vi "Actor Shutdown.vi"(8 "error in (no error)":errorcluster, 11 "IED in":refnum<class "IED.lvclass">) -> (0 "error out":errorcluster, 3 "IED out":refnum<class "IED.lvclass">)   [LabVIEW 2015, in "IED Actor.lvlib" / "IED.lvclass"]
doc: "This VI stops nested actors and sends success or failure to the SCADA Core."
uses:
  IED.lvclass
  IED.lvclass/IED.ctl
  <vilib>/ActorFramework/Message Enqueuer/Message Enqueuer.lvclass/Message Enqueuer.ctl
  <vilib>/ActorFramework/Message Enqueuer/Enqueue.vi
  <vilib>/ActorFramework/Message Priority Queue/Priority Enqueue.vi
  <vilib>/ActorFramework/Stop Msg/Stop Msg.lvclass
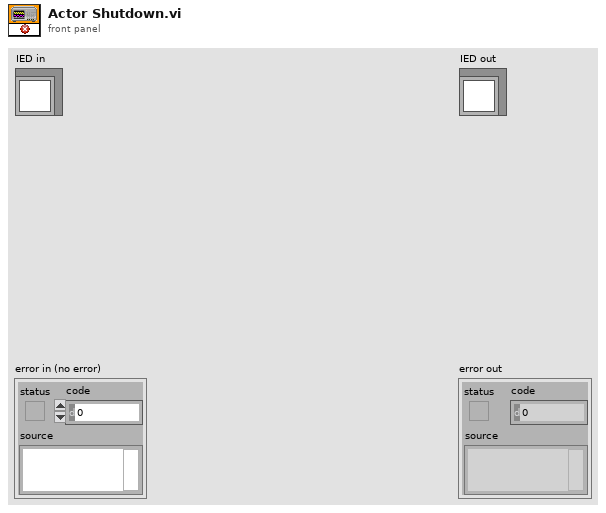
[diagram p1: front panel]
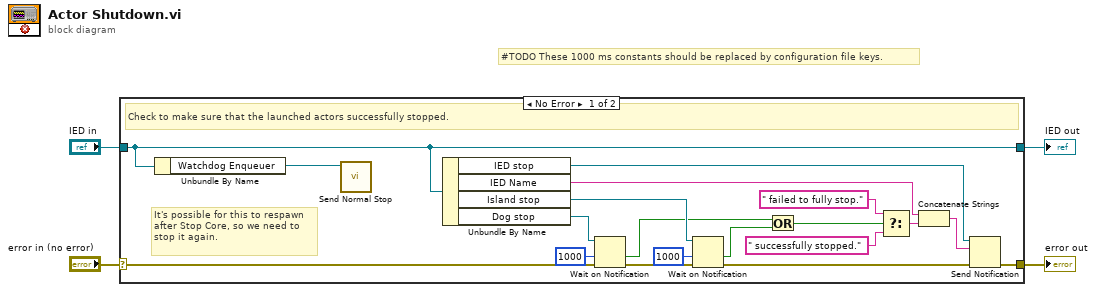
[diagram p0: block diagram]
diagram:
  # "#TODO These 1000 ms constants should be replaced by configuration file keys."
  n1 = case shown="No Error" "error in (no error)" {
    selector: "error in (no error)" -> [w23 w25]
    tunnel: [w14 w25] -> w3
    tunnel: [w6 w24] -> w1
    tunnel: "IED in" -> [w6 w24]
    frame No Error {
      # "It's possible for this to respawn after Stop Core, so we need to stop it again."
      # "Check to make sure that the launched actors successfully stopped."
      n2 = Unbundle By Name(w6) -> ("Watchdog Enqueuer"=w5:refnum<class "Message Enqueuer.lvclass">)
      n3 = call <vilib>:"Send Normal Stop.vi"("Message Enqueuer"=w5) -> ()  [unwired: 10 in, 1 out]
      n4 = Unbundle By Name(w6) -> ("IED stop"=w13:refnum<notifier>, "IED Name"=w8:string, "Island stop"=w19:refnum<notifier>, "Dog stop"=w22:refnum<notifier>)
      n5 = Wait on Notification(notifier=w22, timeout in ms (-1)=1000, error in (no error)=w23) -> (timed out?=w17:bool, error out=w18:errorcluster)  [unwired: 1 in, 2 out]
      n6 = Wait on Notification(notifier=w19, timeout in ms (-1)=1000, error in (no error)=w18) -> (timed out?=w16:bool, error out=w15:errorcluster)  [unwired: 1 in, 2 out]
      n7 = Or(x=w17, y=w16) -> (x .or. y?=w12:bool)
      n8 = Select(t=" failed to fully stop." ("notification"), s=w12, f=" successfully stopped." ("notification")) -> (s? t:f=w9:string)
      n9 = Concatenate Strings(w8, w9) -> (w7:string)
      n10 = Send Notification(notification=w7, notifier=w13, error in (no error)=w15) -> (error out=w14:errorcluster)  [unwired: 1 out]
    }
    frame Error {
    }
  }
  "error out" <- w3
  "IED out" <- w1
